vi "calcHorizontalRadius.vi"(1 "Y Coordinate":i32=238, 2 "X Coordinate":i32=322, 3 "Source Image":T1(plugin-control)) -> (0 "mean radius":dbl)   [LabVIEW 2009, in "ImageAnalysis.lvlib"]
uses:
  ImageAnalysis.lvlib
  <vilib>/vision/NI_Vision_Development_Module.lvlib
panel:
  out "radius(pos)":i32
  out "Pixel Value (U8) 2":u8
  out "radius(neg)":i32
  out "Pixel Value (U8)":u8
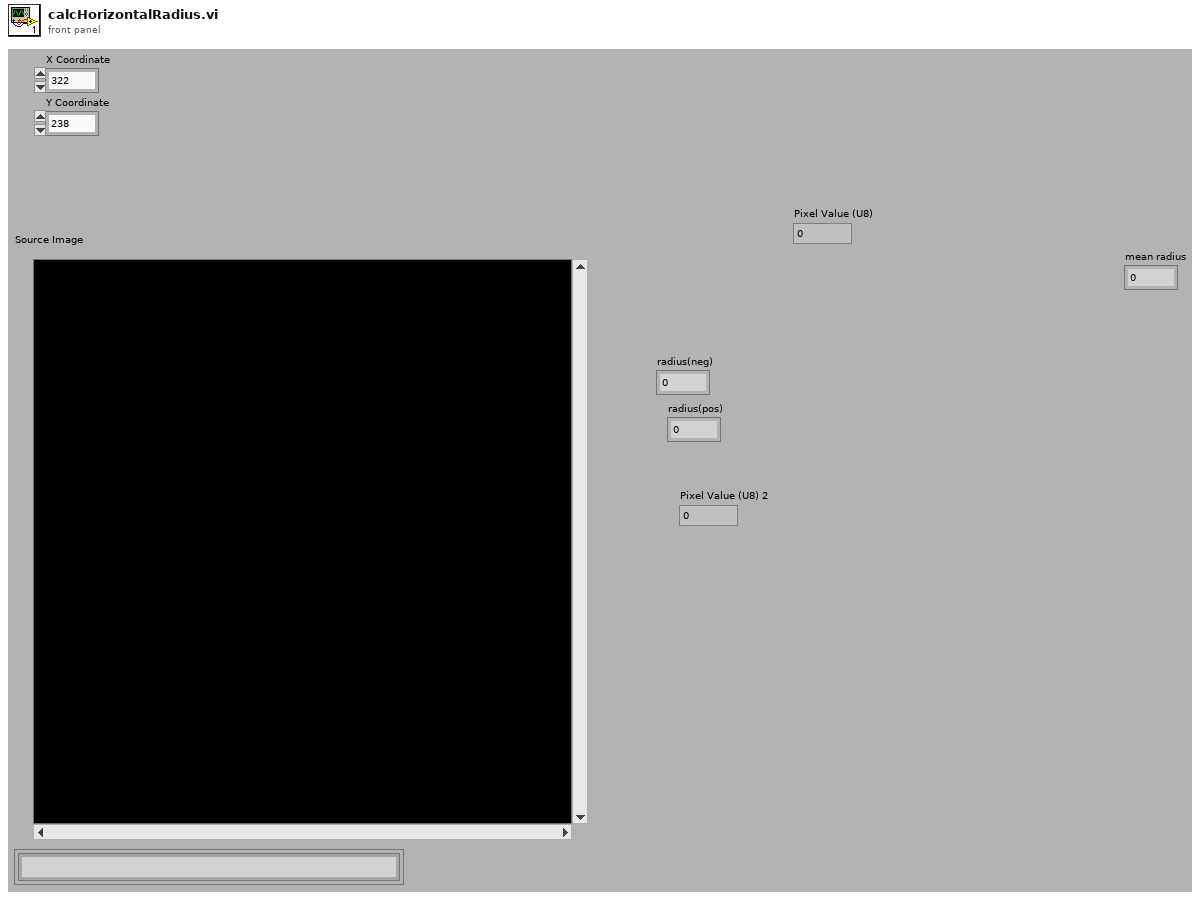
[diagram p1: front panel]
types:
  T1 = typedef "IMAQ Image.ctl" = refnum<image>
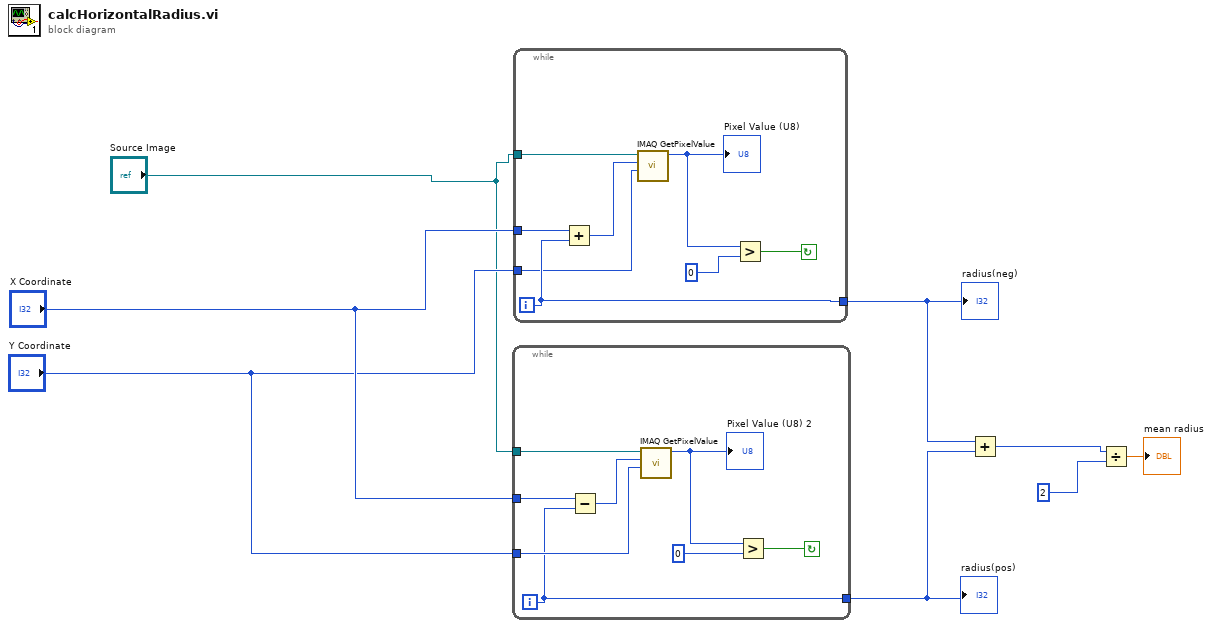
[diagram p0: block diagram]
diagram:
  n1 = while {
    tunnel: "Source Image" -> [w16]
    tunnel: [w9] -> w8
    tunnel: "X Coordinate" -> [w11]
    tunnel: "Y Coordinate" -> [w10]
    i -> [w9]
    stop <- w13 continue-if-true
    n2 = Subtract(x=w11, y=w9) -> (x-y=w12:i32)
    n3 = call "IMAQ GetPixelValue"("Image"=w16, "X Coordinate"=w12, "Y Coordinate"=w10) -> ("Pixel Value (U8)"=w15:u8)  [unwired: 3 in, 4 out]
    "Pixel Value (U8) 2" <- w15
    n4 = Greater?(x=w15, y=u8 0) -> (0:w13:bool)
  }
  "radius(pos)" <- w8
  n5 = while {
    tunnel: "Source Image" -> [w24]
    tunnel: [w19] -> w7
    tunnel: "X Coordinate" -> [w20]
    tunnel: "Y Coordinate" -> [w17]
    i -> [w19]
    stop <- w21 continue-if-true
    n6 = Add(x=w20, y=w19) -> (x+y=w18:i32)
    n7 = call "IMAQ GetPixelValue"("Image"=w24, "X Coordinate"=w18, "Y Coordinate"=w17) -> ("Pixel Value (U8)"=w23:u8)  [unwired: 3 in, 4 out]
    "Pixel Value (U8)" <- w23
    n8 = Greater?(x=w23, y=u8 0) -> (0:w21:bool)
  }
  "radius(neg)" <- w7
  n9 = Add(x=w7, y=w8) -> (x+y=w6:i32)
  n10 = Divide(x=w6, y=2) -> (x/y=→"mean radius":dbl)
